vi "Get ContentInfo.vi"(8 "error in (no error)":errorcluster, 11 "HttpHeaders_Content in":refnum<class "HttpHeaders_Content.lvclass">) -> (0 "error out":errorcluster, 1 "Length":i64, 2 "MediaType":string, 3 "HttpHeaders_Content out":refnum<class "HttpHeaders_Content.lvclass">)   [LabVIEW 2018, in "HttpClient_NET.lvlib" / "HttpHeaders_Content.lvclass"]
doc: "<b> </b> <b> </b>\nHttpClient_NET\nJustin Young - Viviota\nCopyright (c) 2021\nLicense: BSD"
uses:
  HttpHeaders_Content.lvclass
  C:/Viviota/Projects/R&D/__OpenSource/VIV_HTTP_REST_NET/HTTPHeaders_NET/HttpHeaders_NET.lvclass
  HTTPHeaders_NET/HttpHeaders_NET.lvclass/HttpHeaders_NET.ctl
  Read NET_HttpContentHeaders.vi
  HTTPHeaders_NET/Accessors/Read NET_HttpHeaders.vi
  System.Net.Http
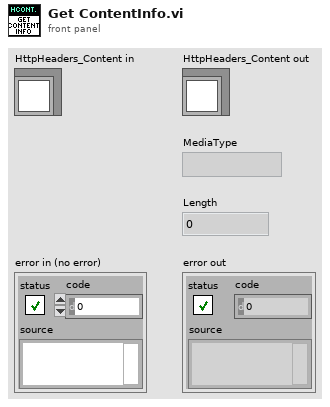
[diagram p1: front panel]
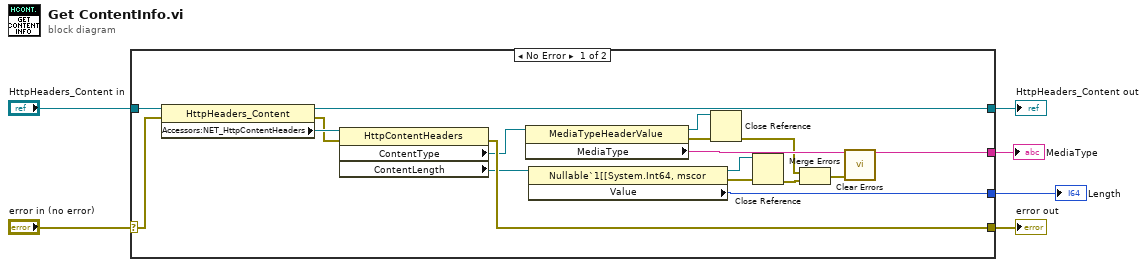
[diagram p0: block diagram]
diagram:
  n1 = case shown="No Error" "error in (no error)" {
    selector: "error in (no error)" -> [w20 w25]
    tunnel: [w18 w25] -> w5
    tunnel: [w22 w24] -> w3
    tunnel: "HttpHeaders_Content in" -> [w23 w24]
    tunnel: [w15 _] -> w2
    tunnel: [w14 _] -> w1
    frame No Error {
      n2 = property class="HttpHeaders_Content"(reference=w23, error in=w20) -> (reference out=w22:refnum<class "HttpHeaders_Content.lvclass">, error out=w19:errorcluster, "Accessors:NET_HttpContentHeaders"=w21:refnum<k24>)
      n3 = property class="HttpContentHeaders"(reference=w21, error in=w19) -> (error out=w18:errorcluster, "ContentType"=w16:refnum<k24>, "ContentLength"=w17:refnum<k24>)  [unwired: 1 out]
      n4 = property class="MediaTypeHeaderValue"(reference=w16) -> (reference out=w12:refnum<k24>, error out=w13:errorcluster, "MediaType"=w15:string)  [unwired: 1 in]
      n5 = property class="Nullable`1[[System.Int64, mscor"(reference=w17) -> (reference out=w10:refnum<k24>, error out=w11:errorcluster, "Value"=w14:i64)  [unwired: 1 in]
      n6 = Close Reference(reference=w12, error in (no error)=w13) -> (error out=w8:errorcluster)
      n7 = Close Reference(reference=w10, error in (no error)=w11) -> (error out=w9:errorcluster)
      n8 = Merge Errors(w8, w9) -> (w7:errorcluster)
      n9 = call <vilib>:"Clear Errors.vi"("error in (no error)"=w7) -> ()  [unwired: 5 in, 2 out]
    }
    frame Error {
    }
  }
  "error out" <- w5
  "HttpHeaders_Content out" <- w3
  "Length" <- w1
  "MediaType" <- w2
